vi "Set StateName.vi"(8 "error in (no error)":errorcluster, 10 "StateName":string, 11 "SMO":refnum<class "SMO.lvclass">) -> (0 "error out":errorcluster, 3 "SMO out":refnum<class "SMO.lvclass">)   [LabVIEW 2019, in "Instrument Attributes.lvlib"]
uses:
  Instrument Attributes.lvlib
  <vilib>/JKI/JKI SMO/SMO/SMO.lvclass
  Attribute.Instrument/Attribute.Instrument.lvclass/Attribute.Instrument.ctl
  SMO.Mediator/SMO.Mediator.lvclass
  Attribute.Instrument/Attribute.Instrument.lvclass
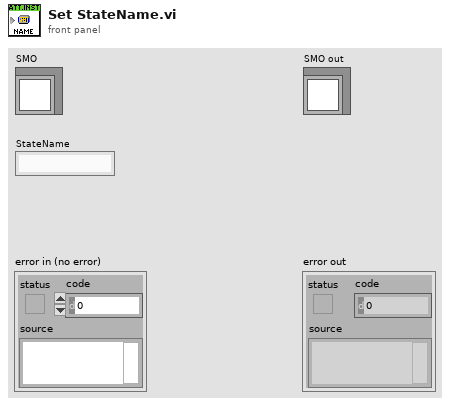
[diagram p1: front panel]
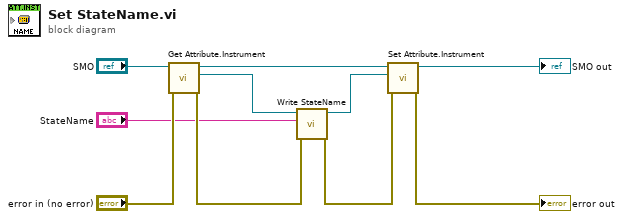
[diagram p0: block diagram]
diagram:
  n1 = call "Get Attribute.Instrument.vi"("error in (no error)"="error in (no error)", "SMO"="SMO") -> ("error out"=w5:errorcluster, "Attribute.Debug"=w2:refnum<class "Attribute.Instrument.lvclass">, "SMO out"=w7:refnum<class "SMO.lvclass">)  [unwired: 7 in]
  n2 = call "Write StateName.vi"("error in (no error)"=w5, "StateName"="StateName", "Attribute.Instrument  in"=w2) -> ("error out"=w3:errorcluster, "Attribute.Instrument out"=w4:refnum<class "Attribute.Instrument.lvclass">)  [unwired: 7 in]
  n3 = call "Set Attribute.Instrument.vi"("error in (no error)"=w3, "Attribute.Debug"=w4, "SMO"=w7) -> ("error out"=→"error out":errorcluster, "SMO out"=→"SMO out":refnum<class "SMO.lvclass">)  [unwired: 7 in]
